vi "sub_potential-field-planning_oscillation-detection.vi"(11 "ixy":cluster{i32, i32}) -> ()   [LabVIEW 2019]
uses:
  Ctrl/cmd_common.ctl
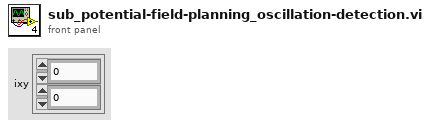
[diagram p1: front panel]
types:
  T1 = typedef "cmd_common.ctl" = enum16{"read", "write"}
  T2 = cluster{"KP":dbl, "ETA":dbl, "AREA_WIDTH":dbl, "Osc_Det_Len":u32}
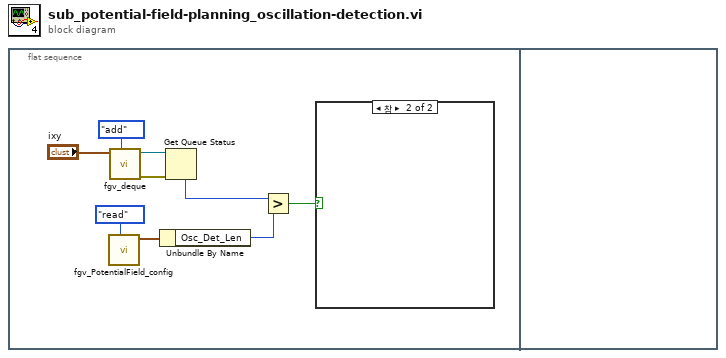
[diagram p0: block diagram]
diagram:
  n1 = flat-sequence {
    frame #0 {
      n2 = call "fgv_PotentialField_config.vi"("cmd"=cmd_common."read") -> ("pf-val out"=w3:T2)  [unwired: 10 in]
      n3 = call "fgv_deque.vi"("cmd"=enum16{"ini", "read", "add", "close"}."add", "start pt"="ixy") -> ("error out"=w6:errorcluster, "queue out"=w7:refnum<queue>)  [unwired: 8 in]
      n4 = Unbundle By Name(w3) -> ("Osc_Det_Len"=w2:u32)
      n5 = Get Queue Status(queue=w7, error in (no error)=w6) -> (# elements in queue=w4:i32)  [unwired: 1 in, 7 out]
      n6 = Greater?(x=w4, y=w2) -> (0:w1:bool)
      n7 = case shown="참" w1 {
        frame False {
        }
        frame True {
        }
      }
    }
    frame #1 {
    }
  }
